vi "PSDATA_Variant To ArrayU32.vi"(9 "error in":errorcluster, 10 "Value":variant) -> (1 "error out":errorcluster, 2 "Value":string, 4 "ArrayU32":u32[](array[numeric]))   [LabVIEW 2016]
doc: "Developer：YDX"
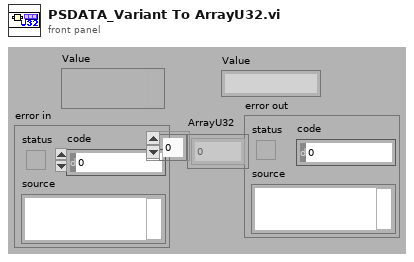
[diagram p1: front panel]
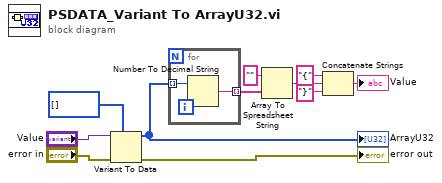
[diagram p0: block diagram]
diagram:
  n1 = Variant To Data(error in="error in", type=u32[] [], Variant="Value") -> (data=w7:u32[], error out=→"error out":errorcluster)
  "ArrayU32" <- w7
  n2 = for {
    tunnel: [w13] -> w2 mode=indexing
    tunnel: w7 -> [w12] mode=indexing
    n3 = Number To Decimal String(number=w12) -> (decimal integer string=w13:string)  [unwired: 1 in]
  }
  n4 = Array To Spreadsheet String(array=w2, 3:"" ("format string")) -> (spreadsheet string=w6:string)  [unwired: 1 in]
  n5 = Concatenate Strings("{" ("string"), w6, "}" ("string")) -> (→"Value":string)
